vi "Receive Signal.vi"(8 "error in":errorcluster, 10 "Frame.Signal":string, 11 "PCAN in":refnum<class "PCAN.lvclass">) -> (0 "error out":errorcluster, 2 "Value":dbl, 3 "PCAN out":refnum<class "PCAN.lvclass">)   [LabVIEW 2023, in "PCAN.lvclass"]
uses:
  PCAN.lvclass
  PCAN.lvclass/PCAN.ctl
  c6e083b5-7be6-46b7-8469-d6fd9ebf7a3d.vi
  c6e083b5-7be6-46b7-8469-d6fd9ebf7a3d.vi/d4db2432-cc9c-482c-8957-dac855435ef6.vi
  c6e083b5-7be6-46b7-8469-d6fd9ebf7a3d.vi/86fbf154-bd7b-49a2-8ab2-a837b2a95f24.vi
  c6e083b5-7be6-46b7-8469-d6fd9ebf7a3d.vi/3b95b01e-1ec2-4565-bcd9-7606a5281010.vi
  c6e083b5-7be6-46b7-8469-d6fd9ebf7a3d.vi/96a08935-737a-44b2-979c-a81d56408f7e.vi
  c6e083b5-7be6-46b7-8469-d6fd9ebf7a3d.vi/d4db2432-cc9c-482c-8957-dac855435ef6.vi/6eaecd13-6e48-4772-a921-b51ebdf84d88.vi
  c6e083b5-7be6-46b7-8469-d6fd9ebf7a3d.vi/d4db2432-cc9c-482c-8957-dac855435ef6.vi/d2d5f2b7-06f4-47f6-971c-049c3fdbb653.vi
  c6e083b5-7be6-46b7-8469-d6fd9ebf7a3d.vi/3b95b01e-1ec2-4565-bcd9-7606a5281010.vi/6eaecd13-6e48-4772-a921-b51ebdf84d88.vi
  c6e083b5-7be6-46b7-8469-d6fd9ebf7a3d.vi/3b95b01e-1ec2-4565-bcd9-7606a5281010.vi/d2d5f2b7-06f4-47f6-971c-049c3fdbb653.vi
  c6e083b5-7be6-46b7-8469-d6fd9ebf7a3d.vi/96a08935-737a-44b2-979c-a81d56408f7e.vi/6eaecd13-6e48-4772-a921-b51ebdf84d88.vi
  c6e083b5-7be6-46b7-8469-d6fd9ebf7a3d.vi/96a08935-737a-44b2-979c-a81d56408f7e.vi/d2d5f2b7-06f4-47f6-971c-049c3fdbb653.vi
  <vilib>/Comparison/Less/Less Functor/Less Functor.lvclass
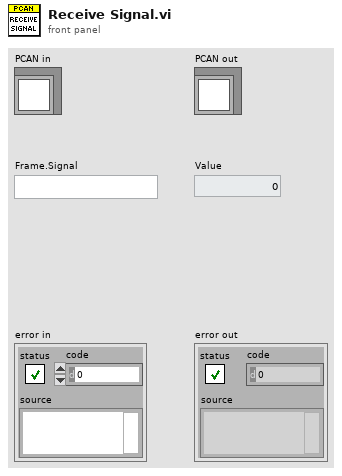
[diagram p1: front panel]
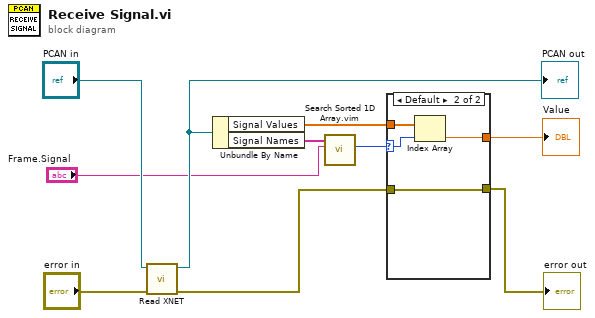
[diagram p0: block diagram]
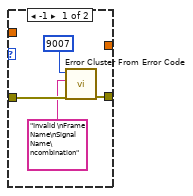
[diagram p2: hidden frame]
diagram:
  n1 = call "Read XNET.vi"("error in"="error in", "PCAN in"="PCAN in") -> ("error out"=w3:errorcluster, "PCAN out"=w8:refnum<class "PCAN.lvclass">)  [unwired: 8 in]
  "PCAN out" <- w8
  n2 = Unbundle By Name(w8) -> ("Signal Values"=w7:dbl[], "Signal Names"=w2:string[])
  n3 = call "Search Sorted 1D Array.vim"("element"="Frame.Signal", "sorted 1D array"=w2) -> ("nearest index"=w1:i32)  [unwired: 8 in, 1 out]
  n4 = case shown="Default" w1 {
    selector: w1 -> [_ w15]
    tunnel: w7 -> [_ w18]
    tunnel: [_ w17] -> w6
    tunnel: w3 -> [w14 w16]
    tunnel: [w13 w16] -> w5
    frame -1 {
      n5 = call <vilib>:"Error Cluster From Error Code.vi"("error in (no error)"=w14, "error message (\"\")"="Invalid \nFrame Name\nSignal Name\ncombination" ("error message (\"\")"), "error code (0)"=9007) -> ("error out"=w13:errorcluster)  [unwired: 6 in]
    }
    frame Default {
      n6 = Index Array(array=w18, index=w15) -> (element=w17:dbl)
    }
  }
  "error out" <- w5
  "Value" <- w6
